vi "Module Cleanup.vi"(8 "error in (no error)":errorcluster, 11 "HTTP Command Bridge in":refnum<class "HTTP Command Bridge.lvclass">) -> (0 "error out":errorcluster, 3 "HTTP Command Bridge out":refnum<class "HTTP Command Bridge.lvclass">)   [LabVIEW 2020, in "Volatus.lvlib" / "HTTP Command Bridge.lvclass"]
uses:
  HTTP Command Bridge.lvclass
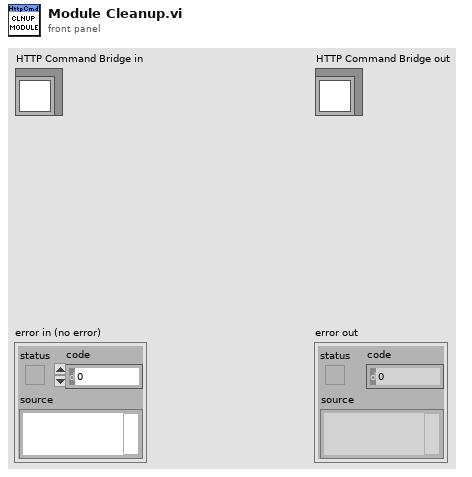
[diagram p1: front panel]
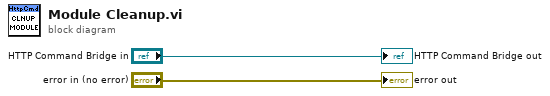
[diagram p0: block diagram]
diagram:
  "error out" <- "error in (no error)"
  "HTTP Command Bridge out" <- "HTTP Command Bridge in"
